vi "PyCom Tests.vi"() -> ()   [LabVIEW 2016]
uses:
  VIs/uPythonX/uPythonX.xctl
panel:
  in  "Tab Control":enum32{"LED", "WiFi", "Timer", "Btn", "BLE"}(tab)=enum."BLE"
  in  "LED":T1(xcontrol)={"VISA Refnum in"="ASRL15::INSTR", "Python Code"="'''\nhttps://docs.pycom.io/gettingstarted/programming/first-project.html\n'''\n\nimport pycom\nimport time\n\npycom.heartbeat(False)\nfor cycles in range(10): # stop after 10 cycles\n    pycom.rgbled(0x007f00) # green\n    time.sleep(1)\n    pycom.rgbled(0x7f7f00) # yellow\n    time.sleep(0.5)\n    pycom.rgbled(0x7f0000) # red\n    time.sleep(1)\n\npycom.rgbled(0)"}
  in  "WiFi":T1(xcontrol)={"VISA Refnum in"="ASRL15::INSTR", "Python Code"="'''\nhttps://docs.pycom.io/tutorials/all/wlan.html\n'''\n\nimport machine\nfrom network import WLAN\nwlan = WLAN(mode=WLAN.STA)\n\nnets = wlan.scan()\n\nnets\n\nfor net in nets:\n    if net.ssid == 'HighPeaks':\n        print('Network found!')\n        wlan.connect(net.ssid, auth=(net.sec, 'password'), timeout=5000)\n        while not wlan.isconnected():\n            machine.idle() # save power while waiting\n        print('WLAN connection succeeded!')\n        break"}
  in  "Timer":T1(xcontrol)={"VISA Refnum in"="ASRL15::INSTR", "Python Code"="'''\nhttps://docs.pycom.io/tutorials/all/timers.html\n'''\n\nfrom machine import Timer\nimport time\n\nchrono = Timer.Chrono()\n\nchrono.start()\ntime.sleep(1.25) # simulate the first lap took 1.25 seconds\nlap = chrono.read() # read elapsed time without stopping\ntime.sleep(1.5)\nchrono.stop()\ntotal = chrono.read()\n\nprint()\nprint(\"\\nthe racer took %f seconds to finish the race\" % total)\nprint(\"  %f seconds in the first lap\" % lap)\nprint(\"  %f seconds in the last lap\" % (total - lap))"}
  in  "Btn":T1(xcontrol)={"VISA Refnum in"="ASRL15::INSTR", "Python Code"="'''\nhttps://github.com/wipy/wipy/blob/master/docs/User_manual_exp_board.pdf\n'''\n\nfrom machine import Pin\nimport time\nimport pycom\n\npycom.heartbeat(False)\n\nled = Pin('G16',Pin.OUT)\nbtn = Pin('G17',Pin.IN,Pin.PULL_UP)\n\n\nled.toggle()\ntime.sleep(1)\nled.value(1)    # 1 is off, 0 is on\n\nbtn.value()    # 1 is off, 0 is on\n\nwhile True:\n     led.value(btn.value())\n     time.sleep(0.2)"}
  in  "BLE":T1(xcontrol)={"VISA Refnum in"="ASRL15::INSTR", "Python Code"="'''\nhttps://docs.pycom.io/firmwareapi/pycom/network/bluetooth/'''\n\nimport ubinascii\nfrom network import Bluetooth\nbluetooth = Bluetooth()\n\nbluetooth.start_scan(10)\nwhile bluetooth.isscanning():\n    adv = bluetooth.get_adv()\n    if adv:\n        # try to get the complete name\n        print(bluetooth.resolve_adv_data(adv.data, Bluetooth.ADV_NAME_SHORT))\n\n        mfg_data = bluetooth.resolve_adv_data(adv.data, Bluetooth.ADV_MANUFACTURER_DATA)\n\n        if mfg_data:\n            # try to get the manufacturer data (Apple's iBeacon data is sent here)\n            print(ubinascii.hexlify(mfg_data))"}
  # "(mac=b'#s\\xc3n\\x9d\\xdc', addr_type=1, adv_type=0, rssi=-97, data=b'\\x02\\x01\\x1b\\x0b\\xffL\\x00\\t\\x06\\x03\\x06\\xc0\\xa8\\x01\\x17\\x00\\x00\\x00\\x00\\x00\\x00\\x00\\x00\\x00\\x00\\x00\\x00\\x00\\x00\\x00\\x00\\x00\\x00\\x00\\x00\\x00\\x00\\x00\\x00\\x00\\x00\\x00\\x00\\x00\\x00\\x00\\x00\\x00\\x00\\x00\\x00\\x00\\x00\\x00\\x00\\x00\\x00\\x00\\x00\\x00\\x00\\x00')"
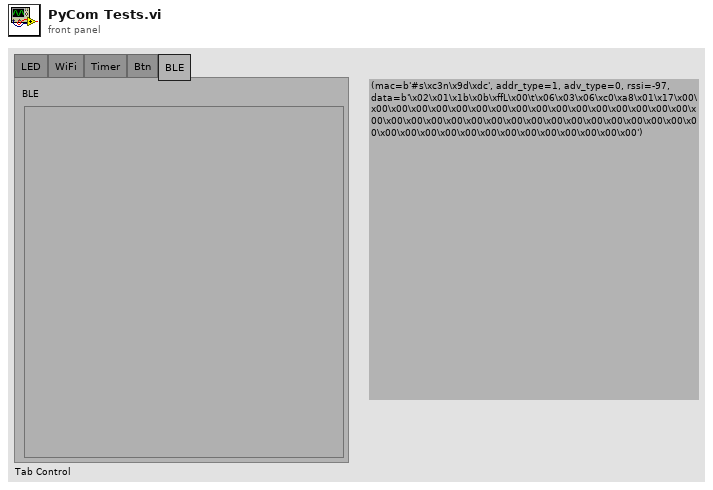
[diagram p1: front panel]
types:
  T1 = cluster{"VISA Refnum in":refnum<visa-resource-name>, "Python Code":string}
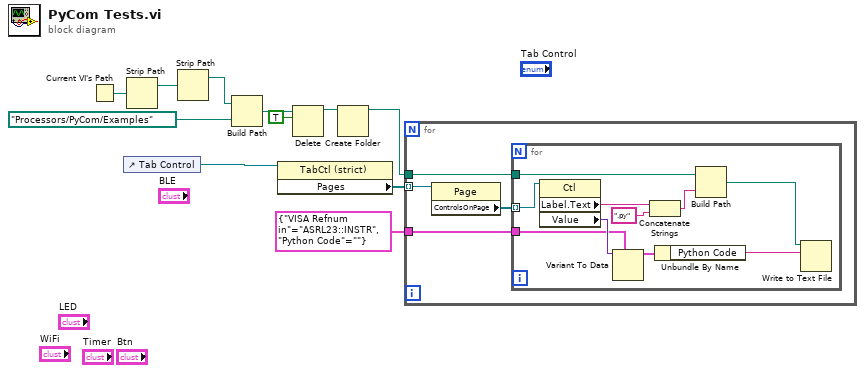
[diagram p0: block diagram]
diagram:
  n1 = Current VI's Path() -> (path=w4:path)
  n2 = control-ref of="Tab Control"() -> (w1:refnum<vi>)
  n3 = Strip Path(path=w4) -> (stripped path=w5:path)  [unwired: 1 out]
  n4 = Strip Path(path=w5) -> (stripped path=w6:path)  [unwired: 1 out]
  n5 = Build Path(base path=w6, name or relative path=path "Processors/PyCom/Examples") -> (appended path=w9:path)
  n6 = property class="TabCtl (strict)"(reference=w1) -> ("Pages"=w2:refnum<vi>[])  [unwired: 1 in, 2 out]
  n7 = Delete(path (use dialog)=w9, entire hierarchy (F)=TRUE) -> (deleted path=w10:path)  [unwired: 3 in, 2 out]
  n8 = Create Folder(path (use dialog)=w10) -> (created path=w11:path)  [unwired: 2 in, 2 out]
  n9 = for {
    tunnel: w2 -> [w15] mode=indexing
    tunnel: T1 {"VISA Refnum in"="ASRL23::INSTR", "Python Code"=""} ("VOC") -> [w13]
    tunnel: w11 -> [w12]
    n10 = property class="Page"(reference=w15) -> ("ControlsOnPage"=w14:refnum<vi>[])  [unwired: 1 in, 2 out]
    n11 = for {
      tunnel: w14 -> [w25] mode=indexing
      tunnel: w13 -> [w23]
      tunnel: w12 -> [w21]
      n12 = property class="Ctl"(reference=w25) -> ("Label.Text"=w20:string, "Value"=w24:variant)  [unwired: 1 in, 2 out]
      n13 = Variant To Data(type=w23, Variant=w24) -> (data=w22:T1)  [unwired: 1 in, 1 out]
      n14 = Concatenate Strings(w20, ".py" ("string")) -> (w19:string)
      n15 = Unbundle By Name(w22) -> ("Python Code"=w16:string)
      n16 = Build Path(base path=w21, name or relative path=w19) -> (appended path=w17:path)
      n17 = Write to Text File(file (use dialog)=w17, text=w16) -> ()  [unwired: 2 in, 3 out]
    }
  }
